vi "Picture_Save_to_matlab.vi"(8 "Input Cluster":T6, 10 "Mode":enum32{"Picture", "Int Trace", "Video"}(ring), 11 "Save":bool) -> ()   [LabVIEW 2009]
uses:
  atmcd32d.llb/AcquisitionMode_mode typedef.ctl
  atmcd32d.llb/ReadMode_mode typedef.ctl
  atmcd32d.llb/TriggerMode_mode typedef.ctl
  atmcd32d.llb/Shutter_type typedef.ctl
  atmcd32d.llb/Shutter_mode typedef.ctl
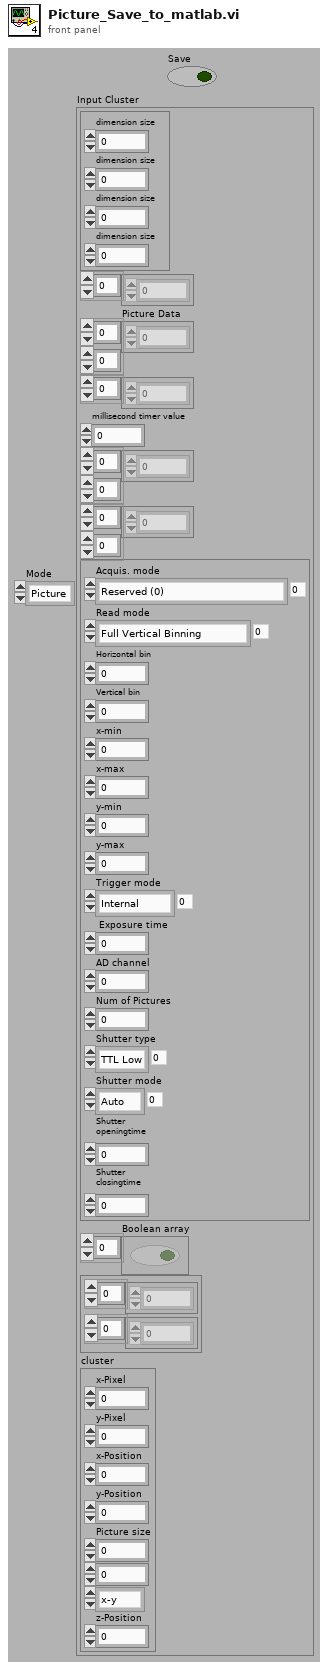
[diagram p1: front panel]
types:
  T1 = typedef "AcquisitionMode_mode typedef.ctl" = enum16{"Reserved (0)", "Single Scan", "Accumulate", "Kinetics", "Fast Kinetics", "Run Till Abort", "Reserved (6)", "Reserved (7)", "Reserved (8)", "Time Delayed Integration"}
  T2 = typedef "ReadMode_mode typedef.ctl" = enum16{"Full Vertical Binning", "Multi-Track", "Random-Track", "Single-Track", "Image"}
  T3 = typedef "TriggerMode_mode typedef.ctl" = enum16{"Internal", "External", "N/A (2)", "N/A (3)", "N/A (4)", "N/A (5)", "External Start"}
  T4 = typedef "Shutter_type typedef.ctl" = enum16{"TTL Low", "TTL High"}
  T5 = typedef "Shutter_mode typedef.ctl" = enum16{"Auto", "Open", "Close"}
  T6 = cluster{cluster{"dimension size":i32, "dimension size":i32, "dimension size":i32, "dimension size":i32}, i32[], "Picture Data":dbl[][], u32[], "millisecond timer value":u32, dbl[][], i32[][], cluster{"Acquis. mode":T1, "Read mode":T2, "Horizontal bin":i32, "Vertical bin":i32, "x-min":i32, "x-max":i32, "y-min":i32, "y-max":i32, "Trigger mode":T3, " Exposure time":sgl, "AD channel":i32, "Num of Pictures":i32, "Shutter type":T4, "Shutter mode":T5, "Shutter\nopeningtime":i32, "Shutter\nclosingtime":i32}, "Boolean array":bool[], cluster{dbl[], dbl[]}, "cluster":cluster{"x-Pixel":u16, "y-Pixel":u16, "x-Position":dbl, "y-Position":dbl, "Picture size":dbl, dbl, enum32{"x-y", "x-z", "y-z"}, "z-Position":dbl}}
  T7 = enum16{"open", "replace", "create", "open or create", "replace or create", "replace or create with confirmation"}
  T8 = cluster{"dimension size":i32, "dimension size":i32, "dimension size":i32, "dimension size":i32}
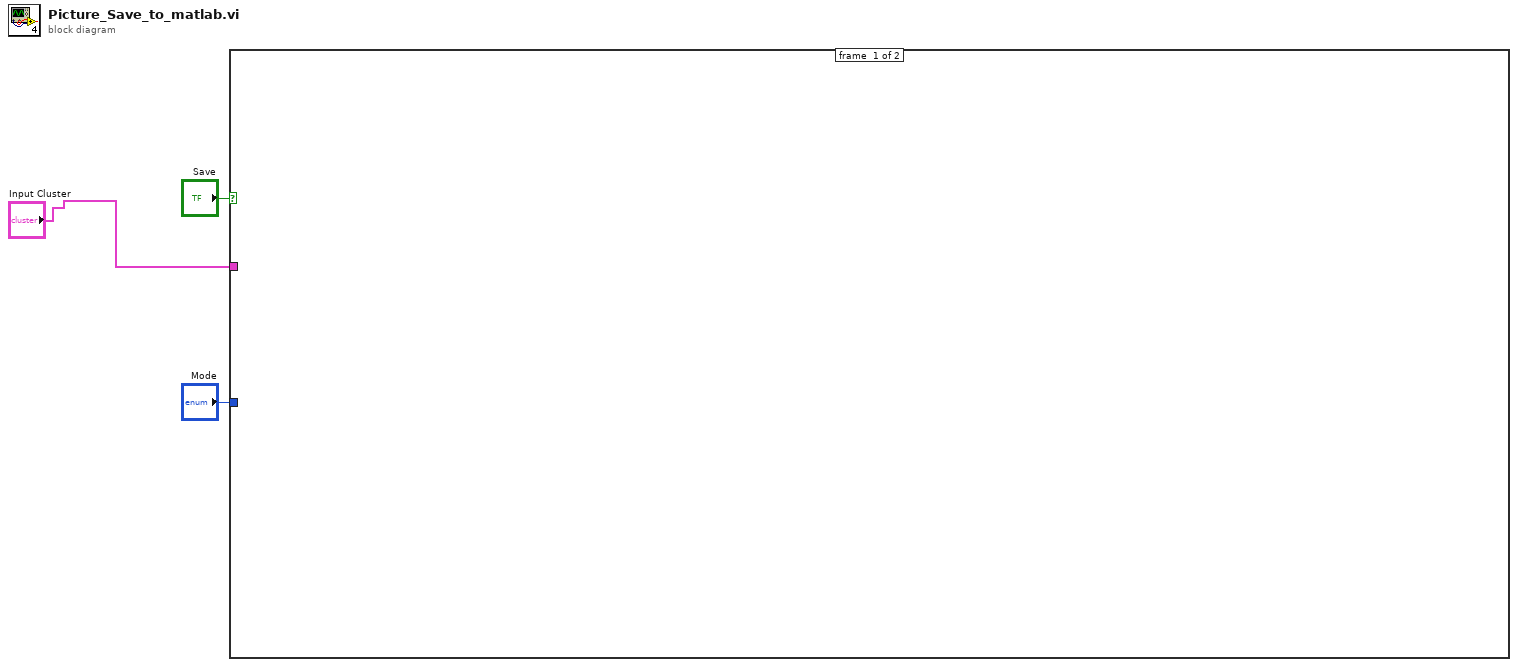
[diagram p0: block diagram]
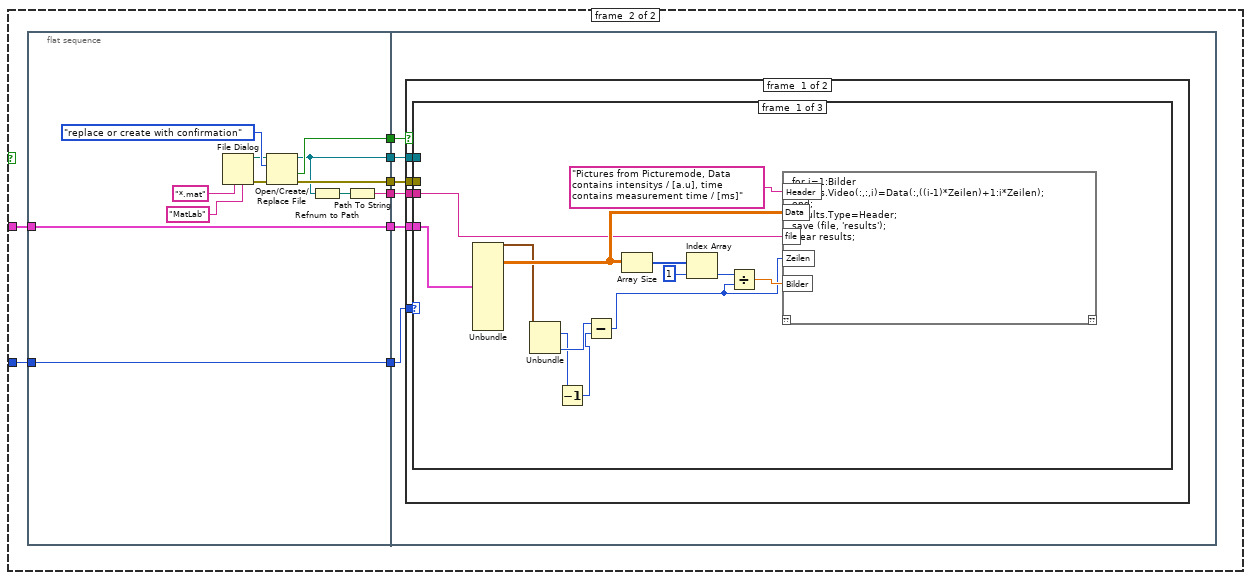
[diagram p2: hidden frame]
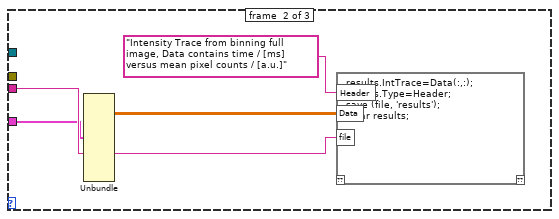
[diagram p3: hidden frame]
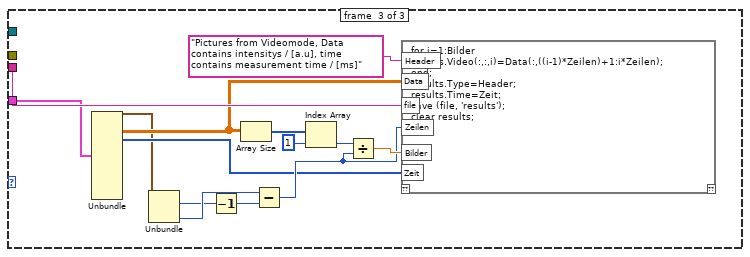
[diagram p4: hidden frame]
diagram:
  n1 = case shown="True" "Save" {
    tunnel: "Mode" -> [_ w11]
    tunnel: "Input Cluster" -> [_ w4]
    frame #0 {
    }
    frame #1 {
      n2 = flat-sequence {
        tunnel: w11 -> [w23]
        tunnel: [w23] -> w10
        tunnel: [w15] -> w9
        tunnel: [w22] -> w8
        tunnel: [w21] -> w7
        tunnel: [w13] -> w6
        tunnel: [w12] -> w5
        tunnel: w4 -> [w12]
        tunnel: w10 -> [w29]
        tunnel: w9 -> [w28]
        tunnel: w8 -> [w26]
        tunnel: w7 -> [w27]
        tunnel: w6 -> [w25]
        tunnel: w5 -> [w24]
        frame #0 {
          n3 = File Dialog(4:"MatLab" ("pattern label"), 6:"*.mat" ("pattern (all files)")) -> (0:w18:errorcluster, 3:w19:path)  [unwired: 1 in, 6 out]
          n4 = Open/Create/Replace File(file path (use dialog)=w19, error in=w18, operation (0:open)=T7."replace or create with confirmation") -> (refnum out=w15:refnum<file>, cancelled=w22:bool, error out=w21:errorcluster)  [unwired: 3 out]
          n5 = Refnum to Path(1:w15) -> (0:w14:path)
          n6 = Path To String(path=w14) -> (string=w13:string)
        }
        frame #1 {
          n7 = case shown="False" w26 {
            tunnel: w29 -> [w34 _]
            tunnel: w28 -> [w33 _]
            tunnel: w27 -> [w32 _]
            tunnel: w25 -> [w31 _]
            tunnel: w24 -> [w30 _]
            frame #0 {
              n8 = case shown="\"Picture\", Default" w34 {
                tunnel: w33 -> [_ _ _]
                tunnel: w32 -> [_ _ _]
                tunnel: w31 -> [w37 w51 w64]
                tunnel: w30 -> [w38 w49 w57]
                frame #0 {
                  n9 = Unbundle(w38) -> (w39:T8, "Picture Data"=w40:dbl[][])  [unwired: 9 out]
                  n10 = Unbundle(w39) -> ("dimension size"=w36:i32, "dimension size"=w41:i32)  [unwired: 2 out]
                  n11 = Decrement(x=w36) -> (x-1=w35:i32)
                  n12 = Subtract(x=w41, y=w35) -> (x-y=w42:i32)
                  n13 = Array Size(array=w40) -> (size(s)=w46:i32[])
                  n14 = Index Array(array=w46, index=1) -> (element=w44:i32)
                  n15 = Divide(x=w44, y=w42) -> (x/y=w43:dbl)
                  n16 = script code="for i=1:Bilder\nresults.Video(:,:,i)=Data(:,((i-1)*Zeilen)+1:i*Zeilen);\nend;\nresults.Type=Header;\nsave (file, 'results');\nclear results;"("file"=w37, "Data"=w40, "Header"="Pictures from Picturemode, Data contains intensitys / [a.u], time contains measurement time / [ms]" ("String"), "Zeilen"=w42, "Bilder"=w43) -> ()  [unwired: 2 out]
                }
                frame #1 {
                  n17 = Unbundle(w49) -> ("Picture Data"=w48:dbl[][])  [unwired: 10 out]
                  n18 = script code="results.IntTrace=Data(:,:);\nresults.Type=Header;\nsave (file, 'results');\nclear results;"("file"=w51, "Data"=w48, "Header"="Intensity Trace from binning full image, Data contains time / [ms] versus mean pixel counts / [a.u.]" ("String")) -> ()  [unwired: 2 out]
                }
                frame #2 {
                  n19 = Unbundle(w57) -> (w54:T8, "Picture Data"=w56:dbl[][], w55:u32[])  [unwired: 8 out]
                  n20 = Unbundle(w54) -> ("dimension size"=w52:i32, "dimension size"=w58:i32)  [unwired: 2 out]
                  n21 = Decrement(x=w52) -> (x-1=w53:i32)
                  n22 = Array Size(array=w56) -> (size(s)=w63:i32[])
                  n23 = Subtract(x=w58, y=w53) -> (x-y=w59:i32)
                  n24 = Index Array(array=w63, index=1) -> (element=w61:i32)
                  n25 = Divide(x=w61, y=w59) -> (x/y=w60:dbl)
                  n26 = script code="for i=1:Bilder\nresults.Video(:,:,i)=Data(:,((i-1)*Zeilen)+1:i*Zeilen);\nend;\nresults.Type=Header;\nresults.Time=Zeit;\nsave (file, 'results');\nclear results;"("file"=w64, "Data"=w56, "Header"="Pictures from Videomode, Data contains intensitys / [a.u], time contains measurement time / [ms]" ("String"), "Zeilen"=w59, "Bilder"=w60, "Zeit"=w55) -> ()  [unwired: 2 out]
                }
              }
            }
            frame #1 {
            }
          }
        }
      }
    }
  }
